vi "EVT Camera Get Param Attr.vi"(9 "attr":cluster{"dataType":i32}, 10 "name":string, 11 "camera":u64) -> (1 "attr out":cluster{"dataType":i32}, 3 "function return":u32(ring))   [LabVIEW 2019, in "EmergentCameraC.lvlib"]
doc: "EMERGENTCAMERAC_API EVT_ERROR EVT_CameraGetParamAttr(Camera_Handle camera, const char* name, struct EvtParamAttribute* attr);"
uses:
  EmergentCameraC.lvlib
  emergentInstall_Windows/win64/eSDK/bin/EmergentCameraC.dll
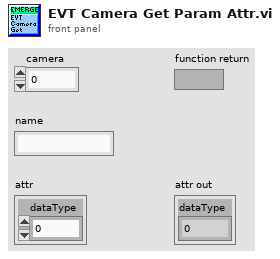
[diagram p1: front panel]
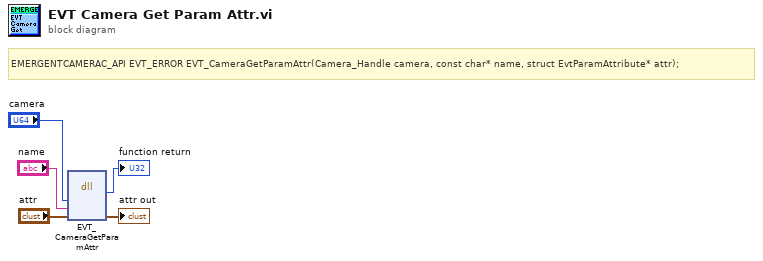
[diagram p0: block diagram]
diagram:
  # "EMERGENTCAMERAC_API EVT_ERROR EVT_CameraGetParamAttr(Camera_Handle camera, const char* name, struct EvtParamAttribute* attr);"
  n1 = dll-call lib="E:/emergent/host-new_QT/emergentInstall_Windows/win64/eSDK/bin/EmergentCameraC.*" fn="EVT_CameraGetParamAttr"("camera"="camera", "name"="name", "attr"="attr") -> (→"function return":u32, "attr"=→"attr out":cluster{"dataType":i32})  [unwired: 5 in, 2 out]
